vi "tracking4.vi"(0 "y":dbl format="%#_13g", 3 "x":dbl format="%#_13g", 5 "reset path":bool, 6 "d":dbl=-0.1 format="%#_13g", 7 "car detection":bool, 8 "x3":dbl=17.0 format="%#_13g", 9 "x2":dbl=8.5 format="%#_13g", 10 "x1":dbl=5.0 format="%#_13g", 11 "xt":dbl) -> (2 "mission":i32)   [LabVIEW 2015]
uses:
  G_ALL.vi
  G_SEN.vi
  G_LCM.vi
panel:
  in  "y 2":dbl=1.0 format="%#_13g"
  out "idx_start":i32
  out "idxx":dbl[](array[numeric])
  out "idx":dbl
  out "dist":dbl[](array[numeric])
  out "y origin":dbl[](array[numeric])
  out "x origin":dbl[](array[numeric])
  out "heading":dbl[](array[numeric])
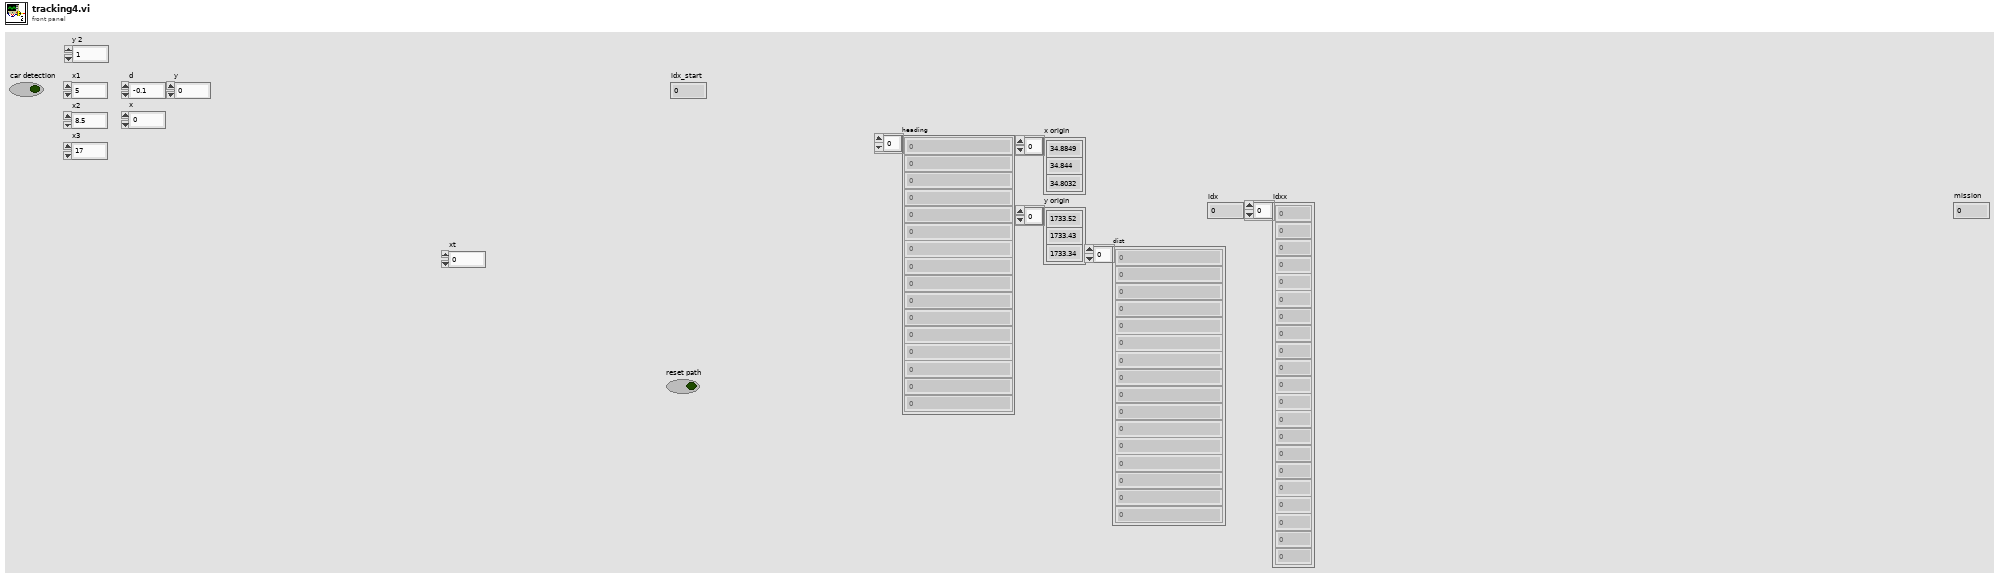
[diagram p1: front panel]
types:
  T1 = cluster{"Steer_input":dbl, "Steer_output":dbl, "VS_des":dbl, "VS_can":dbl, "heading":dbl, "auto":bool, "run":bool, "x":dbl, "y":dbl}
  T2 = cluster{"beep":bool, "duration (msec)":u32, "frequency (Hz)":u32}
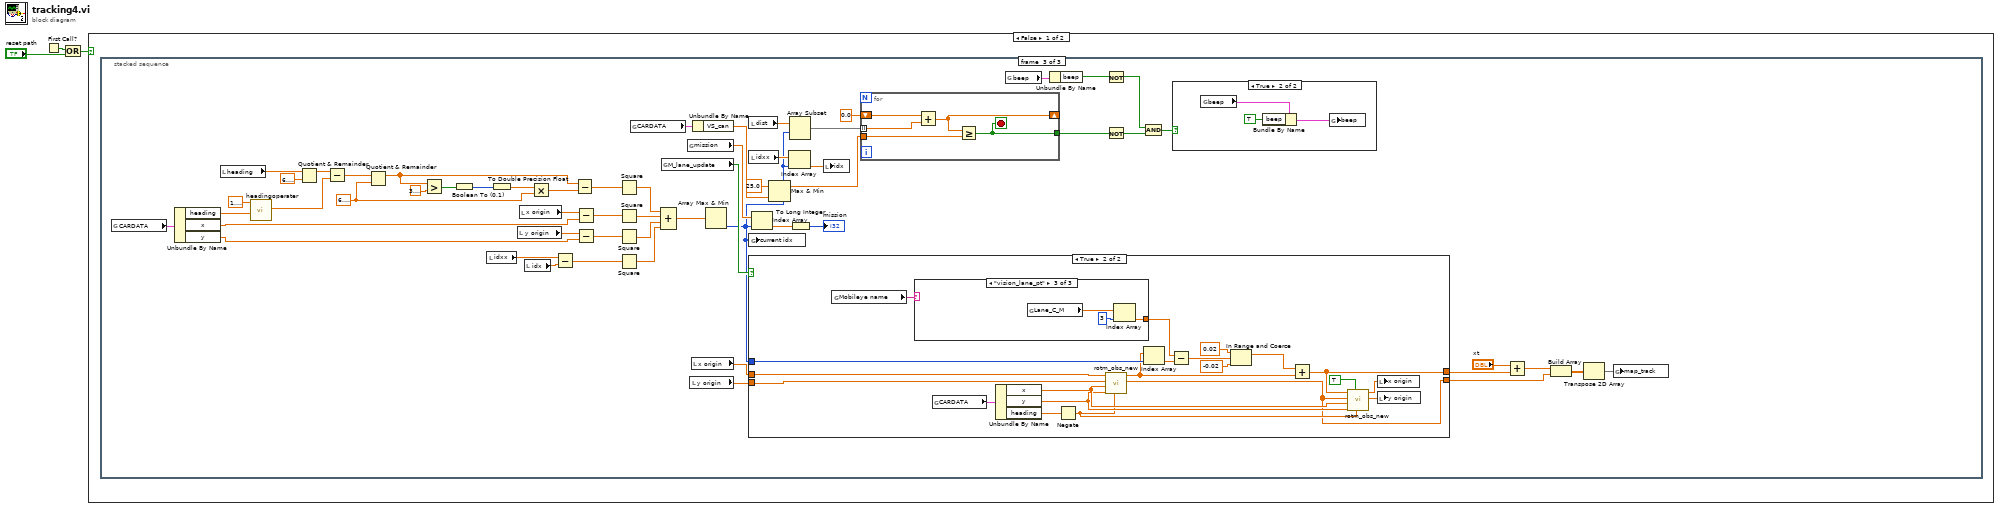
[diagram p0: block diagram]
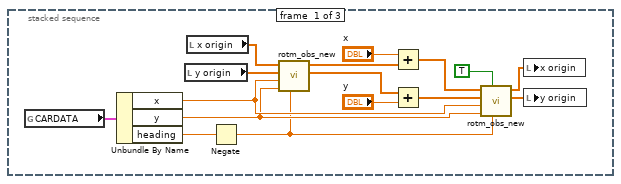
[diagram p2: hidden frame]
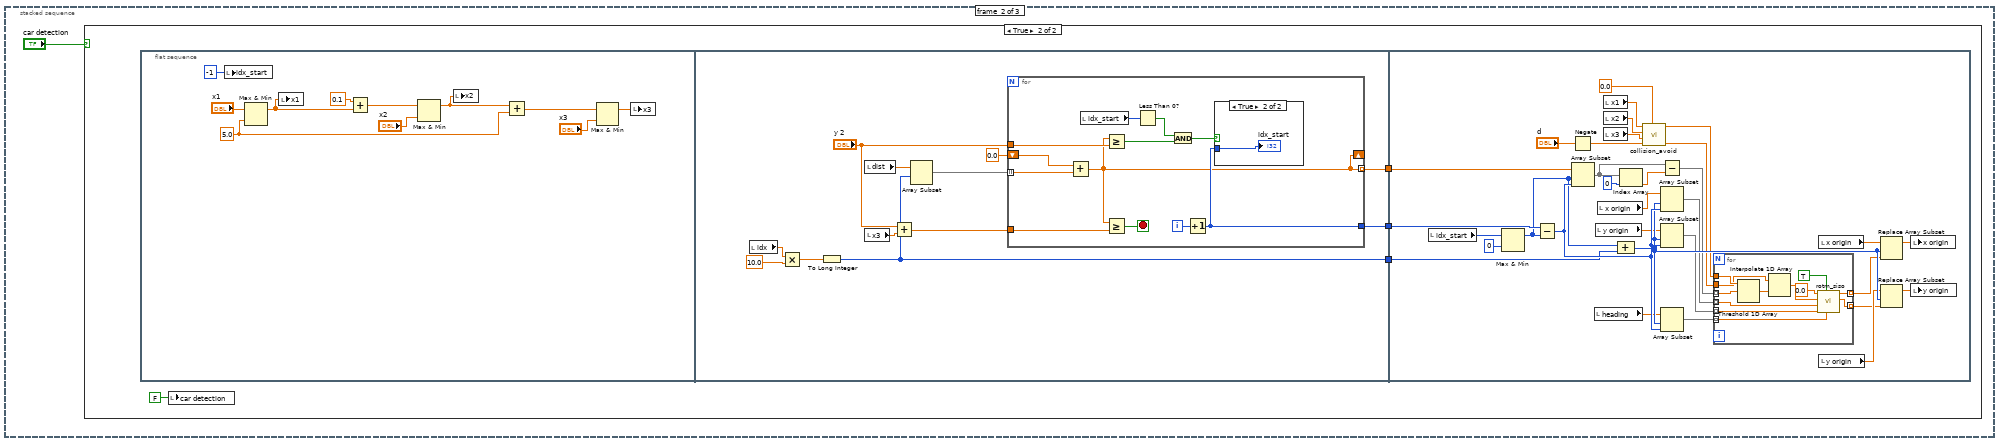
[diagram p3: hidden frame]
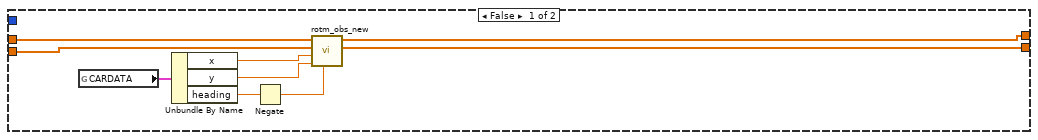
[diagram p7: hidden frame]
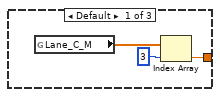
[diagram p8: hidden frame]
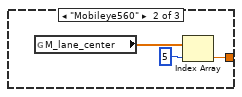
[diagram p9: hidden frame]
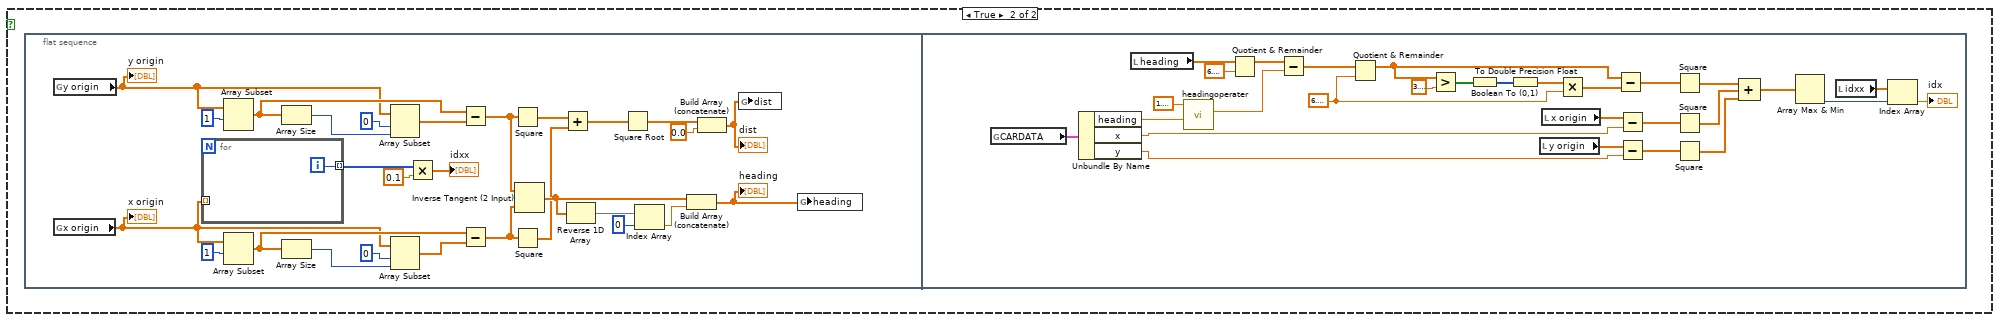
[diagram p10: hidden frame]
diagram:
  n1 = First Call?() -> (First Call?: T/F=w3:bool)
  n2 = Or(x=w3, y="reset path") -> (x .or. y?=w2:bool)
  n3 = case shown="False" w2 {
    frame False {
      n4 = stacked-sequence {
        frame #0 {
          n5 = global read "G_ALL.vi" "CARDATA"() -> (w7:T1)
          n6 = Unbundle By Name(w7) -> ("x"=w12:dbl, "y"=w11:dbl, "heading"=w14:dbl)
          n7 = local read "y origin"() -> (w16:dbl[])
          n8 = local read "x origin"() -> (w15:dbl[])
          n9 = Negate(x=w14) -> (-x=w10:dbl)
          n10 = call "rotm_obs_new.vi"("angle[rad]"=w10, "y0"=w11, "x0"=w12, "y"=w16, "x"=w15) -> ("rot*(y-y0) 2"=w17:dbl[], "rot*(x-x0)"=w6:dbl[])  [unwired: 3 in, 2 out]
          n11 = Add(x="x", y=w6) -> (x+y=w19:dbl[])
          n12 = Add(x=w17, y="y") -> (x+y=w18:dbl[])
          n13 = call "rotm_obs_new.vi"("angle[rad]"=w10, "reverse"=TRUE, "y0"=w11, "x0"=w12, "y"=w18, "x"=w19) -> ("rot*(y-y0) 2"=w8:dbl[], "rot*(x-x0)"=w9:dbl[])  [unwired: 2 in, 2 out]
          n14 = local write "x origin"(w9) -> ()
          n15 = local write "y origin"(w8) -> ()
        }
        frame #1 {
          n16 = case shown="True" "car detection" {
            frame False {
            }
            frame True {
              n17 = flat-sequence {
                tunnel: [w41] -> w23
                tunnel: [w40] -> w22
                tunnel: [w36] -> w21
                tunnel: w21 -> [w63]
                tunnel: w22 -> [w66]
                tunnel: w23 -> [w67]
                frame #0 {
                  w26 = 5.0 ("y")
                  n18 = local write "idx_start"(-1 ("idx_start")) -> ()
                  n19 = Max & Min(x="x1", y=w26) -> (max(x,y)=w32:dbl)  [unwired: 1 out]
                  n20 = local write "x1"(w32) -> ()
                  n21 = Add(x=0.1, y=w32) -> (x+y=w31:dbl)
                  n22 = Max & Min(x=w31, y="x2") -> (max(x,y)=w28:dbl)  [unwired: 1 out]
                  n23 = local write "x2"(w28) -> ()
                  n24 = Add(x=w28, y=w26) -> (x+y=w27:dbl)
                  n25 = Max & Min(x=w27, y="x3") -> (max(x,y)=w29:dbl)  [unwired: 1 out]
                  n26 = local write "x3"(w29) -> ()
                }
                frame #1 {
                  n27 = local read "idx"() -> (w47:dbl)
                  n28 = Multiply(x=w47, y=10.0) -> (x*y=w44:dbl)
                  n29 = To Long Integer(number=w44) -> (32bit integer=w41:i32)
                  n30 = local read "dist"() -> (w45:dbl[])
                  n31 = local read "x3"() -> (w39:dbl)
                  n32 = Add(x="y 2", y=w39) -> (x+y=w38:dbl)
                  n33 = Array Subset(array=w45, index=w41) -> (w43:dbl[])  [unwired: 1 in]
                  n34 = for {
                    tunnel: w43 -> [w59] mode=indexing
                    shift-right: [w48] -> _
                    shift-left: 0.0 -> [w58]
                    tunnel: [w55] -> w40
                    tunnel: w38 -> [w54]
                    tunnel: "y 2" -> [w53]
                    tunnel: [w48] -> w36 mode=indexing
                    i -> [w56]
                    stop <- w57 stop-if-true
                    n35 = Add(x=w58, y=w59) -> (x+y=w48:dbl)
                    n36 = local read "idx_start"() -> (w52:i32)
                    n37 = Greater Or Equal?(x=w48, y=w53) -> (x >= y?=w49:bool)
                    n38 = Greater Or Equal?(x=w48, y=w54) -> (x >= y?=w57:bool)
                    n39 = Less Than 0?(x=w52) -> (x < 0?=w51:bool)
                    n40 = And(x=w51, y=w49) -> (x .and. y?=w50:bool)
                    n41 = Increment(x=w56) -> (x+1=w55:i32)
                    n42 = case shown="True" w50 {
                      tunnel: w55 -> [_ w60]
                      frame False {
                      }
                      frame True {
                        "idx_start" <- w60
                      }
                    }
                  }
                }
                frame #2 {
                  n43 = local read "idx_start"() -> (w65:i32)
                  n44 = Max & Min(x=w65, y=0) -> (max(x,y)=w62:i32)  [unwired: 1 out]
                  n45 = Subtract(x=w66, y=w62) -> (x-y=w91:i32)
                  n46 = Negate(x="d") -> (-x=w69:dbl)
                  n47 = Array Subset(array=w63, index=w62, length=w91) -> (w92:dbl[])
                  n48 = local read "heading"() -> (w75:dbl[])
                  n49 = local read "y origin"() -> (w84:dbl[])
                  n50 = local read "x origin"() -> (w89:dbl[])
                  n51 = local read "x1"() -> (w78:dbl)
                  n52 = local read "x2"() -> (w77:dbl)
                  n53 = local read "x3"() -> (w79:dbl)
                  n54 = Compound Arithmetic op=ADD(w62, w67) -> (w90:i32)
                  n55 = Index Array(array=w92, index=0) -> (element=w87:dbl)
                  n56 = call "collision_avoid.vi"("x0"=0.0, "d"=w69, "x3"=w79, "x2"=w77, "x1"=w78) -> ("y"=w70:dbl[], "x"=w85:dbl[])  [unwired: 5 in]
                  n57 = Subtract(x=w92, y=w87) -> (x-y=w86:dbl[])
                  n58 = Array Subset(array=w89, index=w90, length=w91) -> (w76:dbl[])
                  n59 = Array Subset(array=w84, index=w90, length=w91) -> (w74:dbl[])
                  n60 = Array Subset(array=w75, index=w90, length=w91) -> (w73:dbl[])
                  n61 = for {
                    tunnel: w86 -> [w103] mode=indexing
                    tunnel: w85 -> [w104]
                    tunnel: w70 -> [w102]
                    tunnel: w76 -> [w100] mode=indexing
                    tunnel: w74 -> [w99] mode=indexing
                    tunnel: w73 -> [w98] mode=indexing
                    tunnel: [w97] -> w72 mode=indexing
                    tunnel: [w96] -> w71 mode=indexing
                    n62 = Threshold 1D Array(2:w103, 3:w104) -> (0:w101:dbl)  [unwired: 1 in]
                    n63 = Interpolate 1D Array(1:w101, 2:w102) -> (0:w93:dbl)
                    n64 = call "rotm_siso.vi"("angle[rad]"=w98, "reverse"=TRUE, "y0"=w99, "x0"=w100, "y"=w93, "x"=0.0 ("y")) -> ("y'"=w96:dbl, "x'"=w97:dbl)  [unwired: 4 in]
                  }
                  n65 = local read "x origin"() -> (w83:dbl[])
                  n66 = local read "y origin"() -> (w80:dbl[])
                  n67 = Replace Array Subset(array=w83, new element=w72, index=w90) -> (w82:dbl[])
                  n68 = Replace Array Subset(array=w80, new element=w71, index=w90) -> (w81:dbl[])
                  n69 = local write "x origin"(w82) -> ()
                  n70 = local write "y origin"(w81) -> ()
                }
              }
              n71 = local write "car detection"(FALSE ("Boolean")) -> ()
            }
          }
        }
        frame #2 {
          w147 = 6.283185307179586
          n72 = global read "G_ALL.vi" "CARDATA"() -> (w121:T1)
          n73 = Unbundle By Name(w121) -> ("heading"=w141:dbl, "x"=w162:dbl, "y"=w160:dbl)
          n74 = local read "heading"() -> (w152:dbl[])
          n75 = call "headingoperater.vi"("h1"=w141, "h2"=1.5707963267948966) -> ("h2-h1"=w138:dbl)  [unwired: 8 in, 1 out]
          n76 = Quotient & Remainder(x=w152, y=6.283185307179586) -> (x-y*floor(x/y)=w153:dbl[])  [unwired: 1 out]
          n77 = Subtract(x=w153, y=w138) -> (x-y=w154:dbl[])
          n78 = Quotient & Remainder(x=w154, y=w147) -> (x-y*floor(x/y)=w155:dbl[])  [unwired: 1 out]
          n79 = Greater?(x=w155, y=3.141592653589793) -> (0:w151:bool[])
          n80 = Boolean To (0,1)(Boolean=w151) -> (0, 1=w150:i16[])
          n81 = local read "idxx"() -> (w129:dbl[])
          n82 = To Double Precision Float(number=w150) -> (double precision float=w148:dbl[])
          n83 = local read "y origin"() -> (w159:dbl[])
          n84 = local read "x origin"() -> (w161:dbl[])
          n85 = local read "idx"() -> (w130:dbl)
          n86 = Multiply(x=w148, y=w147) -> (x*y=w149:dbl[])
          n87 = Subtract(x=w129, y=w130) -> (x-y=w128:dbl[])
          n88 = Subtract(x=w155, y=w149) -> (x-y=w146:dbl[])
          n89 = Subtract(x=w161, y=w162) -> (x-y=w144:dbl[])
          n90 = Subtract(x=w159, y=w160) -> (x-y=w145:dbl[])
          n91 = Square(x=w146) -> (x^2=w143:dbl[])
          n92 = Square(x=w144) -> (x^2=w140:dbl[])
          n93 = Square(x=w145) -> (x^2=w139:dbl[])
          n94 = Square(x=w128) -> (x^2=w127:dbl[])
          n95 = global read "G_ALL.vi" "CARDATA"() -> (w120:T1)
          n96 = Compound Arithmetic op=ADD(w143, w140, w139, w127) -> (w142:dbl[])
          n97 = global read "G_SEN.vi" "M_lane_update"() -> (w109:bool)
          n98 = global read "G_ALL.vi" "mission"() -> (w108:dbl[])
          n99 = local read "y origin"() -> (w123:dbl[])
          n100 = local read "x origin"() -> (w133:dbl[])
          n101 = Unbundle By Name(w120) -> ("VS_can"=w119:dbl)
          n102 = Array Max & Min(array=w142) -> (min index (indices)=w107:i32)  [unwired: 3 out]
          n103 = local read "dist"() -> (w137:dbl[])
          n104 = local read "idxx"() -> (w126:dbl[])
          n105 = global write "G_ALL.vi" "current idx"(w107) -> ()
          n106 = case shown="True" w109 {
            tunnel: w133 -> [w170 w190]
            tunnel: w123 -> [w169 w189]
            tunnel: [w166 w183] -> w112
            tunnel: [w168 w186] -> w131
            tunnel: w107 -> [_ w184]
            frame False {
              n107 = global read "G_ALL.vi" "CARDATA"() -> (w167:T1)
              n108 = Unbundle By Name(w167) -> ("x"=w173:dbl, "y"=w172:dbl, "heading"=w174:dbl)
              n109 = Negate(x=w174) -> (-x=w171:dbl)
              n110 = call "rotm_obs_new.vi"("angle[rad]"=w171, "y0"=w172, "x0"=w173, "y"=w169, "x"=w170) -> ("rot*(y-y0) 2"=w168:dbl[], "rot*(x-x0)"=w166:dbl[])  [unwired: 3 in, 2 out]
            }
            frame True {
              n111 = global read "G_LCM.vi" "Mobileye name"() -> (w176:string)
              n112 = case shown="\"vision_lane_pt\"" w176 {
                tunnel: [w196 w199 w202] -> w175
                frame Default {
                  n113 = global read "G_SEN.vi" "Lane_C_M"() -> (w197:dbl[])
                  n114 = Index Array(array=w197, index=3) -> (element=w196:dbl)
                }
                frame "Mobileye560" {
                  n115 = global read "G_SEN.vi" "M_lane_center"() -> (w201:dbl[])
                  n116 = Index Array(array=w201, index=5) -> (element=w199:dbl)
                }
                frame "vision_lane_pt" {
                  n117 = global read "G_SEN.vi" "Lane_C_M"() -> (w203:dbl[])
                  n118 = Index Array(array=w203, index=3) -> (element=w202:dbl)
                }
              }
              n119 = global read "G_ALL.vi" "CARDATA"() -> (w185:T1)
              n120 = Unbundle By Name(w185) -> ("x"=w193:dbl, "y"=w192:dbl, "heading"=w195:dbl)
              n121 = Negate(x=w195) -> (-x=w191:dbl)
              n122 = call "rotm_obs_new.vi"("angle[rad]"=w191, "y0"=w192, "x0"=w193, "y"=w189, "x"=w190) -> ("rot*(y-y0) 2"=w186:dbl[], "rot*(x-x0)"=w181:dbl[])  [unwired: 3 in, 2 out]
              n123 = Index Array(array=w181, index=w184) -> (element=w182:dbl)
              n124 = Subtract(x=w175, y=w182) -> (x-y=w180:dbl)
              n125 = In Range and Coerce(upper limit=0.02, x=w180, lower limit=-0.02) -> (coerced(x)=w177:dbl)  [unwired: 1 out]
              n126 = Add(x=w177, y=w181) -> (x+y=w183:dbl[])
              n127 = call "rotm_obs_new.vi"("angle[rad]"=w191, "reverse"=TRUE, "y0"=w192, "x0"=w193, "y"=w186, "x"=w183) -> ("rot*(y-y0) 2"=w187:dbl[], "rot*(x-x0)"=w188:dbl[])  [unwired: 2 in, 2 out]
              n128 = local write "x origin"(w188) -> ()
              n129 = local write "y origin"(w187) -> ()
            }
          }
          n130 = Index Array(array=w108, index=w107) -> (element=w106:dbl)
          n131 = Max & Min(x=25.0, y=w119) -> (max(x,y)=w113:dbl)  [unwired: 1 out]
          n132 = Index Array(array=w126, index=w107) -> (element=w125:dbl)
          n133 = Array Subset(array=w137, index=w107) -> (w135:dbl[])  [unwired: 1 in]
          n134 = To Long Integer(number=w106) -> (32bit integer=→"mission":i32)
          n135 = local write "idx"(w125) -> ()
          n136 = for {
            tunnel: w135 -> [w209] mode=indexing
            tunnel: w113 -> [w207]
            shift-right: [w208] -> _
            shift-left: 0.0 -> [w206]
            tunnel: [w205] -> w122
            stop <- w205 stop-if-true
            n137 = Add(x=w206, y=w209) -> (x+y=w208:dbl)
            n138 = Greater Or Equal?(x=w208, y=w207) -> (x >= y?=w205:bool)
          }
          n139 = global read "G_ALL.vi" "beep"() -> (w117:T2)
          n140 = Unbundle By Name(w117) -> ("beep"=w116:bool)
          n141 = Not(x=w116) -> (.not. x?=w115:bool)
          n142 = Not(x=w122) -> (.not. x?=w114:bool)
          n143 = And(x=w115, y=w114) -> (x .and. y?=w124:bool)
          n144 = case shown="True" w124 {
            frame False {
            }
            frame True {
              n145 = global read "G_ALL.vi" "beep"() -> (w165:T2)
              n146 = Bundle By Name(cluster=w165, "beep"=TRUE) -> (w164:T2)
              n147 = global write "G_ALL.vi" "beep"(w164) -> ()
            }
          }
          n148 = Add(x="xt", y=w112) -> (x+y=w110:dbl[])
          n149 = Build Array(w110, w131) -> (w132:dbl[][])
          n150 = Transpose 2D Array(2D array=w132) -> (transposed array=w118:dbl[][])
          n151 = global write "G_ALL.vi" "map_track"(w118) -> ()
        }
      }
    }
    frame True {
      n152 = flat-sequence {
        frame #0 {
          n153 = global read "G_ALL.vi" "y origin"() -> (w212:dbl[])
          "y origin" <- w212
          n154 = global read "G_ALL.vi" "x origin"() -> (w213:dbl[])
          "x origin" <- w213
          n155 = for {
            tunnel: w213 -> [_] mode=indexing
            tunnel: [w238] -> w216 mode=indexing
            i -> [w238]
          }
          n156 = Array Subset(array=w212, index=1) -> (w232:dbl[])  [unwired: 1 in]
          n157 = Array Subset(array=w213, index=1) -> (w233:dbl[])  [unwired: 1 in]
          n158 = Array Size(array=w232) -> (size(s)=w229:i32)
          n159 = Array Size(array=w233) -> (size(s)=w236:i32)
          n160 = Array Subset(array=w212, index=0, length=w229) -> (w231:dbl[])
          n161 = Array Subset(array=w213, index=0, length=w236) -> (w234:dbl[])
          n162 = Multiply(x=w216, y=0.1) -> (x*y=→"idxx":dbl[])
          n163 = Subtract(x=w232, y=w231) -> (x-y=w223:dbl[])
          n164 = Subtract(x=w233, y=w234) -> (x-y=w222:dbl[])
          n165 = Square(x=w223) -> (x^2=w221:dbl[])
          n166 = Square(x=w222) -> (x^2=w220:dbl[])
          n167 = Inverse Tangent (2 Input)(1:w222, 2:w223) -> (0:w224:dbl[])
          n168 = Add(x=w221, y=w220) -> (x+y=w219:dbl[])
          n169 = Reverse 1D Array(array=w224) -> (reversed array=w227:dbl[])
          n170 = Square Root(x=w219) -> (sqrt(x)=w218:dbl[])
          n171 = Index Array(array=w227, index=0) -> (element=w225:dbl)
          n172 = Build Array (concatenate)(w224, w225) -> (w210:dbl[])
          "heading" <- w210
          n173 = Build Array (concatenate)(w218, 0.0) -> (w211:dbl[])
          "dist" <- w211
          n174 = global write "G_ALL.vi" "dist"(w211) -> ()
          n175 = global write "G_ALL.vi" "heading"(w210) -> ()
        }
        frame #1 {
          w252 = 6.283185307179586
          n176 = global read "G_ALL.vi" "CARDATA"() -> (w239:T1)
          n177 = Unbundle By Name(w239) -> ("heading"=w246:dbl, "x"=w267:dbl, "y"=w265:dbl)
          n178 = local read "heading"() -> (w257:dbl[])
          n179 = call "headingoperater.vi"("h1"=w246, "h2"=1.5707963267948966) -> ("h2-h1"=w243:dbl)  [unwired: 8 in, 1 out]
          n180 = Quotient & Remainder(x=w257, y=6.283185307179586) -> (x-y*floor(x/y)=w258:dbl[])  [unwired: 1 out]
          n181 = Subtract(x=w258, y=w243) -> (x-y=w259:dbl[])
          n182 = Quotient & Remainder(x=w259, y=w252) -> (x-y*floor(x/y)=w260:dbl[])  [unwired: 1 out]
          n183 = Greater?(x=w260, y=3.141592653589793) -> (0:w256:bool[])
          n184 = Boolean To (0,1)(Boolean=w256) -> (0, 1=w255:i16[])
          n185 = To Double Precision Float(number=w255) -> (double precision float=w253:dbl[])
          n186 = local read "y origin"() -> (w264:dbl[])
          n187 = local read "x origin"() -> (w266:dbl[])
          n188 = Multiply(x=w253, y=w252) -> (x*y=w254:dbl[])
          n189 = Subtract(x=w260, y=w254) -> (x-y=w251:dbl[])
          n190 = Subtract(x=w266, y=w267) -> (x-y=w249:dbl[])
          n191 = Subtract(x=w264, y=w265) -> (x-y=w250:dbl[])
          n192 = Square(x=w251) -> (x^2=w248:dbl[])
          n193 = Square(x=w249) -> (x^2=w245:dbl[])
          n194 = Square(x=w250) -> (x^2=w244:dbl[])
          n195 = Compound Arithmetic op=ADD(w248, w245, w244) -> (w247:dbl[])
          n196 = Array Max & Min(array=w247) -> (min index (indices)=w241:i32)  [unwired: 3 out]
          n197 = local read "idxx"() -> (w242:dbl[])
          n198 = Index Array(array=w242, index=w241) -> (element=→"idx":dbl)
        }
      }
    }
  }
